vi "Initialize CVT.vi"(8 "error in":errorcluster, 11 "Ex Nested in":refnum<class "Ex Nested.lvclass">) -> (0 "error out":errorcluster, 3 "Ex Nested out":refnum<class "Ex Nested.lvclass">)   [LabVIEW 2014, in "Ex Nested.lvclass"]
uses:
  Ex Nested.lvclass
  reusable/Session APIs/CVT/CVT.lvclass
  Ex Nested.lvclass/Ex Nested.ctl
  <userlib>/_Session Fwk/Session - Root.lvclass
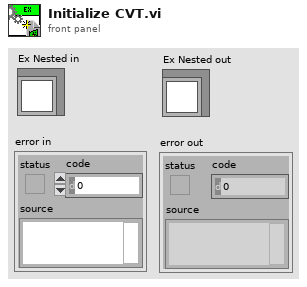
[diagram p1: front panel]
types:
  T1 = typedef "Session - Root.lvclass/Session Handle.ctl" = refnum<data-value>
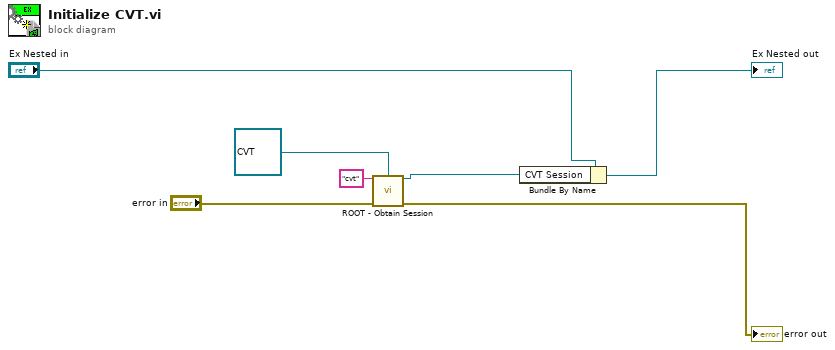
[diagram p0: block diagram]
diagram:
  n1 = call <userlib>:"ROOT - Obtain Session.vi"("Session Name ()"="cvt", "OBJ - Session"=refnum<class "CVT.lvclass"> refnum ("CVT"), "error in (no error)"="error in") -> ("Session Handle"=w2:T1, "error out"=→"error out":errorcluster)  [unwired: 10 in, 1 out]
  n2 = Bundle By Name(cluster="Ex Nested in", "CVT Session"=w2) -> (→"Ex Nested out":refnum<class "Ex Nested.lvclass">)
